vi "HandleObservationSync_002.vi"(8 "error in (no error)":errorcluster, 11 "S4GUI in":refnum<class "S4GUI.lvclass">) -> (0 "error out":errorcluster, 3 "S4GUI out":refnum<class "S4GUI.lvclass">)   [LabVIEW 2018, in "S4GUI.lvclass"] (continued)
              n1509 = Equal?(x=w4372, y=w4362) -> (x = y?=w4370:bool)
              n1510 = call-dynamic "Read stopping.vi"("error in (no error)"=w4365, "Channel in"=w4367) -> ("error out"=w4364:errorcluster, "stopping"=w4363:bool, "Channel out"=w4366:refnum<class "Channel.lvclass">)  [unwired: 7 in]
              n1511 = call-dynamic "Write Channel.vi"("error in (no error)"=w4364, "Channel.lvclass"=w4366, "Acquisition in"=w4375) -> ("error out"=w4377:errorcluster, "Acquisition out"=w4376:refnum<class "Acquisition.lvclass">)  [unwired: 7 in]
            }
          }
          n1512 = call-dynamic "Write AcquisitionC.vi"("error in (no error)"=w4240, "Acquisition.lvclass"=w4238, "S4ACS_GUI in"=w4239) -> ("error out"=w4234:errorcluster, "S4ACS_GUI out"=w4235:refnum<class "S4GUI.lvclass">)  [unwired: 7 in]
          n1513 = call-dynamic "Read AcquisitionD.vi"("error in (no error)"=w4234, "S4ACS_GUI in"=w4235) -> ("error out"=w4218:errorcluster, "Acquisition.lvclass"=w4220:refnum<class "Acquisition.lvclass">, "S4ACS_GUI out"=w4241:refnum<class "S4GUI.lvclass">)  [unwired: 7 in]
          n1514 = call-dynamic "Read enabled.vi"("error in (no error)"=w4218, "Server in"=w4220) -> ("error out"=w4217:errorcluster, "enabled"=w4208:bool, "Server out"=w4219:refnum<class "Acquisition.lvclass">)  [unwired: 7 in]
          n1515 = case shown="True" w4208 {
            tunnel: [w4340 w4356] -> w4243
            tunnel: [w4339 w4355] -> w4242
            tunnel: w4219 -> [w4340 w4354]
            tunnel: w4217 -> [w4339 w4353]
            tunnel: [0 ("State") w4351] -> w4199
            tunnel: w4211 -> [_ w4350]
            tunnel: [TRUE w4349] -> w4209
            tunnel: [FALSE ("stopping") w4342] -> w4195
            frame False {
            }
            frame True {
              n1516 = call-dynamic "Read Channel.vi"("error in (no error)"=w4353, "Acquisition in"=w4354) -> ("error out"=w4348:errorcluster, "Channel.lvclass"=w4347:refnum<class "Channel.lvclass">, "Acquisition out"=w4352:refnum<class "Acquisition.lvclass">)  [unwired: 7 in]
              n1517 = call-dynamic "Read CyclesDone.vi"("error in (no error)"=w4348, "Channel in"=w4347) -> ("error out"=w4344:errorcluster, "CyclesDone"=w4351:u32, "Channel out"=w4346:refnum<class "Channel.lvclass">)  [unwired: 7 in]
              n1518 = Increment(x=w4350) -> (x+1=w4341:u32)
              n1519 = Equal?(x=w4351, y=w4341) -> (x = y?=w4349:bool)
              n1520 = call-dynamic "Read stopping.vi"("error in (no error)"=w4344, "Channel in"=w4346) -> ("error out"=w4343:errorcluster, "stopping"=w4342:bool, "Channel out"=w4345:refnum<class "Channel.lvclass">)  [unwired: 7 in]
              n1521 = call-dynamic "Write Channel.vi"("error in (no error)"=w4343, "Channel.lvclass"=w4345, "Acquisition in"=w4352) -> ("error out"=w4355:errorcluster, "Acquisition out"=w4356:refnum<class "Acquisition.lvclass">)  [unwired: 7 in]
            }
          }
          n1522 = Build Array(w4207, w4206, w4205, w4208) -> (w4204:bool[])
          n1523 = Boolean Array To Number(Boolean array=w4204) -> (number=w4203:u32)
          n1524 = Max & Min(x=w4200, y=w4199) -> (max(x,y)=w4213:u32)  [unwired: 1 out]
          n1525 = Compound Arithmetic op=AND(w4215, w4212, w4210, w4209) -> (w4194:bool)
          n1526 = case shown="15" w4203 {
            tunnel: w4202 -> [w4292 _ w4304 _ w4313 _ w4319 w4325 _ w4331 w4334 _]
            tunnel: w4199 -> [w4291 w4295 w4300 w4307 w4308 w4316 w4318 _ _ _ _ _]
            tunnel: w4201 -> [w4290 w4293 _ _ w4312 w4314 _ w4324 w4328 _ w4333 _]
            tunnel: w4200 -> [w4289 w4294 w4299 w4305 _ _ _ w4323 w4327 w4330 _ _]
            tunnel: [w4285 w4296 w4301 w4306 w4309 w4315 w4317 w4320 w4326 w4329 w4332 TRUE] -> _
            frame 15 {
              # "A,B,C,D ativos"
              n1527 = Equal?(x=w4292, y=w4290) -> (x = y?=w4288:bool)
              n1528 = Equal?(x=w4289, y=w4291) -> (x = y?=w4286:bool)
              n1529 = Equal?(x=w4290, y=w4289) -> (x = y?=w4287:bool)
              n1530 = Compound Arithmetic op=AND(w4288, w4287, w4286) -> (w4285:bool)
            }
            frame 14 {
              # "B,C e,D ativos"
              n1531 = Equal?(x=w4293, y=w4294) -> (x = y?=w4298:bool)
              n1532 = Equal?(x=w4294, y=w4295) -> (x = y?=w4297:bool)
              n1533 = Compound Arithmetic op=AND(w4298, w4297) -> (w4296:bool)
            }
            frame 13 {
              # "A,C e,D ativos"
              n1534 = Equal?(x=w4304, y=w4299) -> (x = y?=w4303:bool)
              n1535 = Equal?(x=w4299, y=w4300) -> (x = y?=w4302:bool)
              n1536 = Compound Arithmetic op=AND(w4303, w4302) -> (w4301:bool)
            }
            frame 12 {
              # "Só C e D ativos"
              n1537 = Equal?(x=w4305, y=w4307) -> (x = y?=w4306:bool)
            }
            frame 11 {
              # "A,B e,D ativos"
              n1538 = Equal?(x=w4313, y=w4312) -> (x = y?=w4311:bool)
              n1539 = Equal?(x=w4312, y=w4308) -> (x = y?=w4310:bool)
              n1540 = Compound Arithmetic op=AND(w4311, w4310) -> (w4309:bool)
            }
            frame 10 {
              # "Só B e D ativos"
              n1541 = Equal?(x=w4314, y=w4316) -> (x = y?=w4315:bool)
            }
            frame 9 {
              # "Só A e D ativos"
              n1542 = Equal?(x=w4319, y=w4318) -> (x = y?=w4317:bool)
            }
            frame 7 {
              # "A,B,C ativos"
              n1543 = Equal?(x=w4325, y=w4324) -> (x = y?=w4322:bool)
              n1544 = Equal?(x=w4324, y=w4323) -> (x = y?=w4321:bool)
              n1545 = Compound Arithmetic op=AND(w4322, w4321) -> (w4320:bool)
            }
            frame 6 {
              # "Só B e C ativos"
              n1546 = Equal?(x=w4328, y=w4327) -> (x = y?=w4326:bool)
            }
            frame 5 {
              # "Só A e C ativos"
              n1547 = Equal?(x=w4331, y=w4330) -> (x = y?=w4329:bool)
            }
            frame 3 {
              # "só A e B ativos"
              n1548 = Equal?(x=w4334, y=w4333) -> (x = y?=w4332:bool)
            }
            frame 0..2, 4, 8, Default {
              # "nenhum ou só 1  \ncanal ativo."
            }
          }
          n1549 = Max & Min(x=w4214, y=w4213) -> (max(x,y)=w4192:u32)  [unwired: 1 out]
          n1550 = Compound Arithmetic op=OR(w4198, w4197, w4196, w4195) -> (w4193:bool)
          n1551 = call-dynamic "Write AcquisitionD.vi"("error in (no error)"=w4242, "Acquisition.lvclass"=w4243, "S4ACS_GUI in"=w4241) -> ("error out"=w4233:errorcluster, "S4ACS_GUI out"=w4190:refnum<class "S4GUI.lvclass">)  [unwired: 7 in]
          n1552 = case shown="True" w4194 {
            tunnel: w4190 -> [w4255 w4273]
            tunnel: [w4261 w4272] -> w4189
            tunnel: w4193 -> [_ w4274]
            tunnel: w4192 -> [_ w4271]
            tunnel: w4191 -> [w4253 w4270]
            frame False {
              # "Aguardando iniciar exposição por 5s"
              n1553 = local read "time1"() -> (w4254:u32)
              n1554 = Tick Count (ms)() -> (millisecond timer value=w4260:u32)
              n1555 = Subtract(x=w4260, y=w4254) -> (x-y=w4257:u32)
              n1556 = To Double Precision Float(number=w4257) -> (double precision float=w4259:dbl)
              n1557 = Less?(x=5000.0 ("y"), y=w4259) -> (x < y?=w4258:bool)
              n1558 = case shown="True" w4258 {
                tunnel: w4255 -> [w4265 w4269]
                tunnel: [w4264 w4268] -> w4261
                tunnel: w4253 -> [w4263 _]
                frame False {
                  # "Volta para esperar ACTIVE."
                  n1559 = Decrement(x=w4263) -> (x-1=w4262:u32)
                  n1560 = Bundle By Name(cluster=w4265, "Obs_state"=w4262) -> (w4264:refnum<class "S4GUI.lvclass">)
                }
                frame True {
                  n1561 = Bundle By Name(cluster=w4269, "Obs_state"=u32 1, "Error Msg"="ERROR: Init Acquisition Timeout. HandleObservationSync.vi - state 327.") -> (w4268:refnum<class "S4GUI.lvclass">)
                }
              }
            }
            frame True {
              # "STOP?"
              # "CIclo Avançou."
              n1562 = case shown="False" w4274 {
                tunnel: w4273 -> [w4278 w4284]
                tunnel: [w4277 w4283] -> w4272
                tunnel: w4271 -> [w4276 w4282]
                tunnel: w4270 -> [_ w4281]
                frame True {
                  # "STOP acionado."
                  n1563 = Bundle By Name(cluster=w4278, "Obs_state"=u32 0, "cyclesDone"=w4276) -> (w4277:refnum<class "S4GUI.lvclass">)
                }
                frame False {
                  # "Vai esperar fim da exposição..."
                  n1564 = Increment(x=w4281) -> (x+1=w4280:u32)
                  n1565 = Increment(x=w4280) -> (x+1=w4279:u32)
                  n1566 = Bundle By Name(cluster=w4284, "Obs_state"=w4279, "cyclesDone"=w4282) -> (w4283:refnum<class "S4GUI.lvclass">)
                }
              }
            }
          }
        }
        frame 328 {
          # "T= canais receberam STOP"
          n1567 = Unbundle By Name(w4444) -> ("cyclesDone"=w4438:u32)
          n1568 = call-dynamic "Read AcquisitionA.vi"("error in (no error)"=w4480, "S4ACS_GUI in"=w4444) -> ("error out"=w4459:errorcluster, "Acquisition.lvclass"=w4460:refnum<class "Acquisition.lvclass">, "S4ACS_GUI out"=w4482:refnum<class "S4GUI.lvclass">)  [unwired: 7 in]
          n1569 = call-dynamic "Read enabled.vi"("error in (no error)"=w4459, "Server in"=w4460) -> ("error out"=w4458:errorcluster, "enabled"=w4434:bool, "Server out"=w4457:refnum<class "Acquisition.lvclass">)  [unwired: 7 in]
          n1570 = case shown="True" w4434 {
            tunnel: w4458 -> [w4631 w4648]
            tunnel: [w4632 w4646] -> w4483
            tunnel: [w4631 w4645] -> w4481
            tunnel: [0 ("State") w4641] -> w4429
            tunnel: w4457 -> [w4632 w4640]
            tunnel: w4438 -> [_ w4639]
            tunnel: [TRUE w4638] -> w4443
            tunnel: [FALSE ("stopping") w4634] -> w4425
            frame False {
            }
            frame True {
              n1571 = call-dynamic "Read Channel.vi"("error in (no error)"=w4648, "Acquisition in"=w4640) -> ("error out"=w4644:errorcluster, "Channel.lvclass"=w4643:refnum<class "Channel.lvclass">, "Acquisition out"=w4647:refnum<class "Acquisition.lvclass">)  [unwired: 7 in]
              n1572 = call-dynamic "Read CyclesDone.vi"("error in (no error)"=w4644, "Channel in"=w4643) -> ("error out"=w4636:errorcluster, "CyclesDone"=w4641:u32, "Channel out"=w4642:refnum<class "Channel.lvclass">)  [unwired: 7 in]
              n1573 = Increment(x=w4639) -> (x+1=w4633:u32)
              n1574 = Equal?(x=w4641, y=w4633) -> (x = y?=w4638:bool)
              n1575 = call-dynamic "Read stopping.vi"("error in (no error)"=w4636, "Channel in"=w4642) -> ("error out"=w4635:errorcluster, "stopping"=w4634:bool, "Channel out"=w4637:refnum<class "Channel.lvclass">)  [unwired: 7 in]
              n1576 = call-dynamic "Write Channel.vi"("error in (no error)"=w4635, "Channel.lvclass"=w4637, "Acquisition in"=w4647) -> ("error out"=w4645:errorcluster, "Acquisition out"=w4646:refnum<class "Acquisition.lvclass">)  [unwired: 7 in]
            }
          }
          n1577 = call-dynamic "Write AcquisitionA.vi"("error in (no error)"=w4481, "Acquisition.lvclass"=w4483, "S4ACS_GUI in"=w4482) -> ("error out"=w4476:errorcluster, "S4ACS_GUI out"=w4475:refnum<class "S4GUI.lvclass">)  [unwired: 7 in]
          n1578 = call "Read AcquisitionB.vi"("error in (no error)"=w4476, "S4ACS_GUI in"=w4475) -> ("error out"=w4453:errorcluster, "Acquisition.lvclass"=w4456:refnum<class "Acquisition.lvclass">, "S4ACS_GUI out"=w4477:refnum<class "S4GUI.lvclass">)  [unwired: 7 in]
          n1579 = call-dynamic "Read enabled.vi"("error in (no error)"=w4453, "Server in"=w4456) -> ("error out"=w4454:errorcluster, "enabled"=w4433:bool, "Server out"=w4455:refnum<class "Acquisition.lvclass">)  [unwired: 7 in]
          n1580 = case shown="True" w4433 {
            tunnel: w4454 -> [w4610 w4627]
            tunnel: w4455 -> [w4611 w4626]
            tunnel: [0 ("State") w4619] -> w4428
            tunnel: [w4610 w4625] -> w4474
            tunnel: [w4611 w4624] -> w4473
            tunnel: w4438 -> [_ w4618]
            tunnel: [TRUE w4617] -> w4439
            tunnel: [FALSE ("stopping") w4613] -> w4424
            frame False {
            }
            frame True {
              n1581 = call-dynamic "Read Channel.vi"("error in (no error)"=w4627, "Acquisition in"=w4626) -> ("error out"=w4622:errorcluster, "Channel.lvclass"=w4623:refnum<class "Channel.lvclass">, "Acquisition out"=w4620:refnum<class "Acquisition.lvclass">)  [unwired: 7 in]
              n1582 = call-dynamic "Read CyclesDone.vi"("error in (no error)"=w4622, "Channel in"=w4623) -> ("error out"=w4615:errorcluster, "CyclesDone"=w4619:u32, "Channel out"=w4621:refnum<class "Channel.lvclass">)  [unwired: 7 in]
              n1583 = Increment(x=w4618) -> (x+1=w4612:u32)
              n1584 = Equal?(x=w4619, y=w4612) -> (x = y?=w4617:bool)
              n1585 = call-dynamic "Read stopping.vi"("error in (no error)"=w4615, "Channel in"=w4621) -> ("error out"=w4614:errorcluster, "stopping"=w4613:bool, "Channel out"=w4616:refnum<class "Channel.lvclass">)  [unwired: 7 in]
              n1586 = call-dynamic "Write Channel.vi"("error in (no error)"=w4614, "Channel.lvclass"=w4616, "Acquisition in"=w4620) -> ("error out"=w4625:errorcluster, "Acquisition out"=w4624:refnum<class "Acquisition.lvclass">)  [unwired: 7 in]
            }
          }
          n1587 = Max & Min(x=w4429, y=w4428) -> (max(x,y)=w4442:u32)  [unwired: 1 out]
          n1588 = call "Write AcquisitionB.vi"("error in (no error)"=w4474, "Acquisition.lvclass"=w4473, "S4ACS_GUI in"=w4477) -> ("error out"=w4466:errorcluster, "S4ACS_GUI out"=w4465:refnum<class "S4GUI.lvclass">)  [unwired: 7 in]
          n1589 = call-dynamic "Read AcquisitionC.vi"("error in (no error)"=w4466, "S4ACS_GUI in"=w4465) -> ("error out"=w4450:errorcluster, "Acquisition.lvclass"=w4452:refnum<class "Acquisition.lvclass">, "S4ACS_GUI out"=w4468:refnum<class "S4GUI.lvclass">)  [unwired: 7 in]
          n1590 = call-dynamic "Read enabled.vi"("error in (no error)"=w4450, "Server in"=w4452) -> ("error out"=w4449:errorcluster, "enabled"=w4432:bool, "Server out"=w4451:refnum<class "Acquisition.lvclass">)  [unwired: 7 in]
          n1591 = case shown="True" w4432 {
            tunnel: [w4589 w4606] -> w4469
            tunnel: [w4590 w4605] -> w4467
            tunnel: w4449 -> [w4589 w4602]
            tunnel: w4451 -> [w4590 w4603]
            tunnel: [0 ("State") w4601] -> w4427
            tunnel: w4438 -> [_ w4600]
            tunnel: [TRUE w4599] -> w4437
            tunnel: [FALSE ("stopping") w4592] -> w4423
            frame False {
            }
            frame True {
              n1592 = call-dynamic "Read Channel.vi"("error in (no error)"=w4602, "Acquisition in"=w4603) -> ("error out"=w4598:errorcluster, "Channel.lvclass"=w4597:refnum<class "Channel.lvclass">, "Acquisition out"=w4604:refnum<class "Acquisition.lvclass">)  [unwired: 7 in]
              n1593 = call-dynamic "Read CyclesDone.vi"("error in (no error)"=w4598, "Channel in"=w4597) -> ("error out"=w4594:errorcluster, "CyclesDone"=w4601:u32, "Channel out"=w4596:refnum<class "Channel.lvclass">)  [unwired: 7 in]
              n1594 = Increment(x=w4600) -> (x+1=w4591:u32)
              n1595 = Equal?(x=w4601, y=w4591) -> (x = y?=w4599:bool)
              n1596 = call-dynamic "Read stopping.vi"("error in (no error)"=w4594, "Channel in"=w4596) -> ("error out"=w4593:errorcluster, "stopping"=w4592:bool, "Channel out"=w4595:refnum<class "Channel.lvclass">)  [unwired: 7 in]
              n1597 = call-dynamic "Write Channel.vi"("error in (no error)"=w4593, "Channel.lvclass"=w4595, "Acquisition in"=w4604) -> ("error out"=w4606:errorcluster, "Acquisition out"=w4605:refnum<class "Acquisition.lvclass">)  [unwired: 7 in]
            }
          }
          n1598 = call-dynamic "Write AcquisitionC.vi"("error in (no error)"=w4469, "Acquisition.lvclass"=w4467, "S4ACS_GUI in"=w4468) -> ("error out"=w4463:errorcluster, "S4ACS_GUI out"=w4464:refnum<class "S4GUI.lvclass">)  [unwired: 7 in]
          n1599 = call-dynamic "Read AcquisitionD.vi"("error in (no error)"=w4463, "S4ACS_GUI in"=w4464) -> ("error out"=w4446:errorcluster, "Acquisition.lvclass"=w4448:refnum<class "Acquisition.lvclass">, "S4ACS_GUI out"=w4470:refnum<class "S4GUI.lvclass">)  [unwired: 7 in]
          n1600 = call-dynamic "Read enabled.vi"("error in (no error)"=w4446, "Server in"=w4448) -> ("error out"=w4445:errorcluster, "enabled"=w4435:bool, "Server out"=w4447:refnum<class "Acquisition.lvclass">)  [unwired: 7 in]
          n1601 = case shown="True" w4435 {
            tunnel: [w4569 w4585] -> w4472
            tunnel: [w4568 w4584] -> w4471
            tunnel: w4447 -> [w4569 w4583]
            tunnel: w4445 -> [w4568 w4582]
            tunnel: [0 ("State") w4580] -> w4426
            tunnel: w4438 -> [_ w4579]
            tunnel: [TRUE w4578] -> w4436
            tunnel: [FALSE ("stopping") w4571] -> w4422
            frame False {
            }
            frame True {
              n1602 = call-dynamic "Read Channel.vi"("error in (no error)"=w4582, "Acquisition in"=w4583) -> ("error out"=w4577:errorcluster, "Channel.lvclass"=w4576:refnum<class "Channel.lvclass">, "Acquisition out"=w4581:refnum<class "Acquisition.lvclass">)  [unwired: 7 in]
              n1603 = call-dynamic "Read CyclesDone.vi"("error in (no error)"=w4577, "Channel in"=w4576) -> ("error out"=w4573:errorcluster, "CyclesDone"=w4580:u32, "Channel out"=w4575:refnum<class "Channel.lvclass">)  [unwired: 7 in]
              n1604 = Increment(x=w4579) -> (x+1=w4570:u32)
              n1605 = Equal?(x=w4580, y=w4570) -> (x = y?=w4578:bool)
              n1606 = call-dynamic "Read stopping.vi"("error in (no error)"=w4573, "Channel in"=w4575) -> ("error out"=w4572:errorcluster, "stopping"=w4571:bool, "Channel out"=w4574:refnum<class "Channel.lvclass">)  [unwired: 7 in]
              n1607 = call-dynamic "Write Channel.vi"("error in (no error)"=w4572, "Channel.lvclass"=w4574, "Acquisition in"=w4581) -> ("error out"=w4584:errorcluster, "Acquisition out"=w4585:refnum<class "Acquisition.lvclass">)  [unwired: 7 in]
            }
          }
          n1608 = Build Array(w4434, w4433, w4432, w4435) -> (w4431:bool[])
          n1609 = Boolean Array To Number(Boolean array=w4431) -> (number=w4430:u32)
          n1610 = Max & Min(x=w4427, y=w4426) -> (max(x,y)=w4441:u32)  [unwired: 1 out]
          n1611 = Compound Arithmetic op=AND(w4443, w4439, w4437, w4436) -> (w4420:bool)
          n1612 = case shown="15" w4430 {
            tunnel: w4429 -> [w4491 _ w4503 _ w4512 _ w4518 w4524 _ w4530 w4533 _]
            tunnel: w4426 -> [w4490 w4494 w4499 w4506 w4507 w4515 w4517 _ _ _ _ _]
            tunnel: w4428 -> [w4489 w4492 _ _ w4511 w4513 _ w4523 w4527 _ w4532 _]
            tunnel: w4427 -> [w4488 w4493 w4498 w4504 _ _ _ w4522 w4526 w4529 _ _]
            tunnel: [w4484 w4495 w4500 w4505 w4508 w4514 w4516 w4519 w4525 w4528 w4531 TRUE] -> _
            frame 15 {
              # "A,B,C,D ativos"
              n1613 = Equal?(x=w4491, y=w4489) -> (x = y?=w4487:bool)
              n1614 = Equal?(x=w4488, y=w4490) -> (x = y?=w4485:bool)
              n1615 = Equal?(x=w4489, y=w4488) -> (x = y?=w4486:bool)
              n1616 = Compound Arithmetic op=AND(w4487, w4486, w4485) -> (w4484:bool)
            }
            frame 14 {
              # "B,C e,D ativos"
              n1617 = Equal?(x=w4492, y=w4493) -> (x = y?=w4497:bool)
              n1618 = Equal?(x=w4493, y=w4494) -> (x = y?=w4496:bool)
              n1619 = Compound Arithmetic op=AND(w4497, w4496) -> (w4495:bool)
            }
            frame 13 {
              # "A,C e,D ativos"
              n1620 = Equal?(x=w4503, y=w4498) -> (x = y?=w4502:bool)
              n1621 = Equal?(x=w4498, y=w4499) -> (x = y?=w4501:bool)
              n1622 = Compound Arithmetic op=AND(w4502, w4501) -> (w4500:bool)
            }
            frame 12 {
              # "Só C e D ativos"
              n1623 = Equal?(x=w4504, y=w4506) -> (x = y?=w4505:bool)
            }
            frame 11 {
              # "A,B e,D ativos"
              n1624 = Equal?(x=w4512, y=w4511) -> (x = y?=w4510:bool)
              n1625 = Equal?(x=w4511, y=w4507) -> (x = y?=w4509:bool)
              n1626 = Compound Arithmetic op=AND(w4510, w4509) -> (w4508:bool)
            }
            frame 10 {
              # "Só B e D ativos"
              n1627 = Equal?(x=w4513, y=w4515) -> (x = y?=w4514:bool)
            }
            frame 9 {
              # "Só A e D ativos"
              n1628 = Equal?(x=w4518, y=w4517) -> (x = y?=w4516:bool)
            }
            frame 7 {
              # "A,B,C ativos"
              n1629 = Equal?(x=w4524, y=w4523) -> (x = y?=w4521:bool)
              n1630 = Equal?(x=w4523, y=w4522) -> (x = y?=w4520:bool)
              n1631 = Compound Arithmetic op=AND(w4521, w4520) -> (w4519:bool)
            }
            frame 6 {
              # "Só B e C ativos"
              n1632 = Equal?(x=w4527, y=w4526) -> (x = y?=w4525:bool)
            }
            frame 5 {
              # "Só A e C ativos"
              n1633 = Equal?(x=w4530, y=w4529) -> (x = y?=w4528:bool)
            }
            frame 3 {
              # "só A e B ativos"
              n1634 = Equal?(x=w4533, y=w4532) -> (x = y?=w4531:bool)
            }
            frame 0..2, 4, 8, Default {
              # "nenhum ou só 1  \ncanal ativo."
            }
          }
          n1635 = Max & Min(x=w4442, y=w4441) -> (max(x,y)=w4440:u32)  [unwired: 1 out]
          n1636 = Compound Arithmetic op=OR(w4425, w4424, w4423, w4422) -> (w4421:bool)
          n1637 = call-dynamic "Write AcquisitionD.vi"("error in (no error)"=w4471, "Acquisition.lvclass"=w4472, "S4ACS_GUI in"=w4470) -> ("error out"=w4461:errorcluster, "S4ACS_GUI out"=w4462:refnum<class "S4GUI.lvclass">)  [unwired: 7 in]
          n1638 = case shown="True" w4420 {
            tunnel: w4462 -> [w4545 w4555]
            tunnel: [w4544 w4554] -> w4479
            tunnel: w4478 -> [_ w4553]
            tunnel: w4440 -> [_ w4552]
            tunnel: w4421 -> [_ w4551]
            frame False {
              # "Aguardando avanço do ciclo."
              n1639 = local read "time307"() -> (w4535:u32)
              n1640 = Tick Count (ms)() -> (millisecond timer value=w4543:u32)
              n1641 = Subtract(x=w4543, y=w4535) -> (x-y=w4540:u32)
              n1642 = call-dynamic "GetGreatestCube.vi"("S4GUI in"=w4545) -> ("S4GUI out"=w4536:refnum<class "S4GUI.lvclass">, "greatest (ms)"=w4538:dbl)  [unwired: 8 in, 1 out]
              n1643 = To Double Precision Float(number=w4540) -> (double precision float=w4542:dbl)
              n1644 = Add(x=5000.0 ("y"), y=w4538) -> (x+y=w4537:dbl)
              n1645 = Less?(x=w4537, y=w4542) -> (x < y?=w4541:bool)
              n1646 = case shown="True" w4541 {
                tunnel: w4536 -> [w4546 w4550]
                tunnel: [w4546 w4549] -> w4544
                frame False {
                }
                frame True {
                  n1647 = Bundle By Name(cluster=w4550, "Obs_state"=u32 1, "Error Msg"="ERROR: Acquisition Timeout. HandleObservationSync.vi - state 328.") -> (w4549:refnum<class "S4GUI.lvclass">)
                }
              }
            }
            frame True {
              # "Ciclo avançou."
              # "STOP?"
              n1648 = case shown="False" w4551 {
                tunnel: w4555 -> [w4559 w4564]
                tunnel: [w4558 w4563] -> w4554
                tunnel: w4553 -> [_ w4561]
                tunnel: w4552 -> [w4557 w4560]
                frame True {
                  n1649 = Bundle By Name(cluster=w4559, "Obs_state"=u32 0, "cyclesDone"=w4557) -> (w4558:refnum<class "S4GUI.lvclass">)
                }
                frame False {
                  n1650 = Increment(x=w4561) -> (x+1=w4562:u32)
                  n1651 = Bundle By Name(cluster=w4564, "Obs_state"=w4562, "cyclesDone"=w4560) -> (w4563:refnum<class "S4GUI.lvclass">)
                }
              }
            }
          }
        }
        frame 329 {
          n1652 = disable-structure shown="Enabled" {
            disable-tunnel: w4653 -> [w4667 w4673]
            disable-tunnel: w4652 -> [w4666 w4680]
            disable-tunnel: [w4665 w4680] -> w4651
            disable-tunnel: [w4663 w4681] -> w4650
            disable-tunnel: w4649 -> [_ w4674]
            frame Disabled {
              n1653 = call-dynamic "Read ciclos.vi"("error in (no error)"=w4666, "S4ACS_GUI in"=w4667) -> ("error out"=w4655:errorcluster, "ciclos"=w4660:u32, "S4ACS_GUI out"=w4668:refnum<class "S4GUI.lvclass">)  [unwired: 7 in]
              n1654 = Decrement(x=w4660) -> (x-1=w4654:u32)
              n1655 = Greater Than 0?(x=w4654) -> (x > 0?=w4661:bool)
              n1656 = case shown="False" w4661 {
                selector: w4661 -> [w4670 w4672]
                tunnel: w4654 -> [_ w4671]
                tunnel: [w4670 w4672] -> w4659
                tunnel: [u32 0 w4671] -> w4656
                frame False {
                }
                frame True {
                }
              }
              n1657 = Select(t=u32 323, s=w4659, f=u32 0) -> (s? t:f=w4662:u32)
              n1658 = call-dynamic "Write ciclos.vi"("error in (no error)"=w4655, "ciclos"=w4656, "S4ACS_GUI in"=w4668) -> ("error out"=w4665:errorcluster, "S4ACS_GUI out"=w4664:refnum<class "S4GUI.lvclass">)  [unwired: 7 in]
              n1659 = Bundle By Name(cluster=w4664, "Obs_state"=w4662) -> (w4663:refnum<class "S4GUI.lvclass">)
            }
            frame Enabled {
              n1660 = Unbundle By Name(w4673) -> ("TotalCiclos"=w4683:u32, "cyclesDone"=w4682:u32)
              n1661 = Subtract(x=w4683, y=w4682) -> (x-y=w4676:u32)
              n1662 = Greater Than 0?(x=w4676) -> (x > 0?=w4679:bool)
              n1663 = disable-structure shown="Enabled" {
                disable-tunnel: [w4685 u32 325 ("t")] -> w4675
                disable-tunnel: w4674 -> [w4684 _]
                frame Disabled {
                  n1664 = Increment(x=w4684) -> (x+1=w4685:u32)
                }
                frame Enabled {
                }
              }
              n1665 = Select(t=w4675, s=w4679, f=u32 0) -> (s? t:f=w4678:u32)
              n1666 = Bundle By Name(cluster=w4673, "ciclos"=w4676, "Obs_state"=w4678) -> (w4681:refnum<class "S4GUI.lvclass">)
            }
          }
        }
        frame 350 {
          n1667 = flat-sequence {
            tunnel: w4688 -> [w4728]
            tunnel: [w4728] -> w4687
            frame #0 {
              n1668 = Tick Count (ms)() -> (millisecond timer value=→"timer350":u32)
            }
          }
          n1669 = call "Read Instrument.lvclass.vi"("error in (no error)"=w4687, "S4ACS_GUI in"=w4723) -> ("error out"=w4726:errorcluster, "Instrument.lvclass"=w4727:refnum<class "Instrument.lvclass">, "S4ACS_GUI out"=w4724:refnum<class "S4GUI.lvclass">)  [unwired: 7 in]
          n1670 = call "Read WPROT.vi"("error in (no error)"=w4726, "Instrument in"=w4727) -> ("error out"=w4716:errorcluster, "Opt_Selector.lvclass"=w4717:refnum<class "Opt_Selector.lvclass">, "Instrument out"=w4725:refnum<class "Instrument.lvclass">)  [unwired: 7 in]
          n1671 = call-dynamic "getTargetPos.vi"("error in (no error)"=w4716, "Opt_Selector in"=w4717) -> ("error out"=w4715:errorcluster, "Target Pos"=w4695:u16, "Opt_Selector out"=w4714:refnum<class "Opt_Selector.lvclass">)  [unwired: 7 in]
          n1672 = Build Array(-1.0 ("element"), 0.0 ("element"), 22.5 ("element"), 45.0 ("element"), 67.5 ("element"), 90.0 ("element"), 112.5 ("element"), 135.0 ("element"), 157.5 ("element"), 180.0 ("element"), 202.5 ("element"), 225.0 ("element"), 247.5 ("element"), 270.0 ("element"), 292.5 ("element"), 315.0 ("element"), 337.5 ("element")) -> (w4707:dbl[])
          n1673 = Index Array(array=w4707, index=w4695) -> (element=w4694:dbl)
          n1674 = case shown="0, Default" w4695 {
            selector: w4695 -> [_ w4757]
            tunnel: w4725 -> [w4737 w4745]
            tunnel: [w4737 w4745] -> w4690
            tunnel: [w4734 w4744] -> w4689
            tunnel: w4720 -> [_ w4759]
            tunnel: [u32 352 w4758] -> w4719
            tunnel: w4715 -> [w4735 w4753]
            tunnel: w4714 -> [w4736 w4752]
            tunnel: w4694 -> [_ w4747]
            tunnel: [w4732 w4746] -> w4691
            frame 0, Default {
              # "Terminou uma sequência.\nRecupera as posições em SEQ e desvia para 311 para verificar se há mais ciclos."
              # "Recupera a sequencia anterior para o caso \nde repetição da sequencia (sem precisar clicar \nnas posicoes desejadas novamente)."
              n1675 = call-dynamic "Read sequencia_ant.vi"("error in (no error)"=w4735, "Opt_Selector in"=w4736) -> ("error out"=w4731:errorcluster, "sequencia_ant"=w4730:u16, "Opt_Selector out"=w4733:refnum<class "Opt_Selector.lvclass">)  [unwired: 7 in]
              n1676 = call-dynamic "Write sequencia.vi"("error in (no error)"=w4731, "sequencia"=w4730, "Opt_Selector in"=w4733) -> ("error out"=w4734:errorcluster, "Opt_Selector out"=w4732:refnum<class "Opt_Selector.lvclass">)  [unwired: 7 in]
            }
            frame 1..16 {
              # "Espera até 40 x 0.25s (= 10s) para\nmecanismo entrar em READY"
              n1677 = Number To Decimal String(number=w4757) -> (decimal integer string=w4756:string)  [unwired: 1 in]
              n1678 = Concatenate Strings("WP" ("string"), w4756) -> (w4754:string)
              n1679 = call "Write target name.vi"("error in (no error)"=w4753, "target name"=w4754, "Optics in"=w4752) -> ("error out"=w4750:errorcluster, "Optics out"=w4751:refnum<class "Opt_Selector.lvclass">)  [unwired: 7 in]
              n1680 = call "Write target.vi"("error in (no error)"=w4750, "target"=w4747, "Optics in"=w4751) -> ("error out"=w4749:errorcluster, "Optics out"=w4748:refnum<class "Opt_Selector.lvclass">)  [unwired: 7 in]
              n1681 = call-dynamic "Read State Machine.vi"("error in (no error)"=w4749, "Device in"=w4748) -> ("error out"=w4761:errorcluster, "State Machine.lvclass"=w4763:refnum<class "State Machine.lvclass">, "Device out"=w4760:refnum<class "Opt_Selector.lvclass">)  [unwired: 7 in]
              n1682 = Increment(x=w4759) -> (x+1=w4758:u32)
              n1683 = call "Next State.vi"("error in (no error)"=w4761, "New_State"=1, "State Machine in"=w4763) -> ("error out"=w4741:errorcluster, "State Machine out"=w4743:refnum<class "State Machine.lvclass">)  [unwired: 7 in]
              n1684 = call-dynamic "Write Timer.vi"("error in (no error)"=w4741, "Timer"=u32 40, "State Machine in"=w4743) -> ("error out"=w4740:errorcluster, "State Machine out"=w4742:refnum<class "State Machine.lvclass">)  [unwired: 7 in]
              n1685 = call-dynamic "Write State Machine.vi"("error in (no error)"=w4740, "State Machine.lvclass"=w4742, "Device in"=w4760) -> ("error out"=w4744:errorcluster, "Device out"=w4746:refnum<class "Opt_Selector.lvclass">)  [unwired: 7 in]
            }
          }
          n1686 = call "Write WPROT.vi"("error in (no error)"=w4689, "Opt_Selector.lvclass"=w4691, "Instrument in"=w4690) -> ("error out"=w4693:errorcluster, "Instrument out"=w4692:refnum<class "Instrument.lvclass">)  [unwired: 7 in]
          n1687 = call "Write Instrument.lvclass.vi"("error in (no error)"=w4693, "Instrument.lvclass"=w4692, "S4ACS_GUI in"=w4724) -> ("error out"=w4722:errorcluster, "S4ACS_GUI out"=w4721:refnum<class "S4GUI.lvclass">)  [unwired: 7 in]
          n1688 = Bundle By Name(cluster=w4721, "Obs_state"=w4719) -> (w4718:refnum<class "S4GUI.lvclass">)
        }
        frame 351 {
          # "Espera terminar o movimento da lamina para disparar a aquisição\ndos canais ativos.\n\nOV 20230424: Não precisa mais atualizar o valor de WPPOS com o\ncomando WRITE_HEADER porque o ACS já recebeu a sequência de\nposições da lâmina."
          n1689 = flat-sequence {
            tunnel: w4774 -> [w4793]
            tunnel: [w4793] -> w4773
            frame #0 {
              n1690 = Tick Count (ms)() -> (millisecond timer value=w4792:u32)
              "timer351" <- w4792
              n1691 = local read "time1"() -> (w4791:u32)
              n1692 = Subtract(x=w4792, y=w4791) -> (x-y=→"delay wp 2":u32)
            }
          }
          n1693 = call "Read Instrument.lvclass.vi"("error in (no error)"=w4773, "S4ACS_GUI in"=w4783) -> ("error out"=w4788:errorcluster, "Instrument.lvclass"=w4789:refnum<class "Instrument.lvclass">, "S4ACS_GUI out"=w4785:refnum<class "S4GUI.lvclass">)  [unwired: 7 in]
          n1694 = call "Read WPROT.vi"("error in (no error)"=w4788, "Instrument in"=w4789) -> ("error out"=w4780:errorcluster, "Opt_Selector.lvclass"=w4779:refnum<class "Opt_Selector.lvclass">, "Instrument out"=w4787:refnum<class "Instrument.lvclass">)  [unwired: 7 in]
          n1695 = call-dynamic "Read State Machine.vi"("error in (no error)"=w4780, "Device in"=w4779) -> ("error out"=w4781:errorcluster, "State Machine.lvclass"=w4782:refnum<class "State Machine.lvclass">, "Device out"=w4777:refnum<class "Opt_Selector.lvclass">)  [unwired: 7 in]
          n1696 = call-dynamic "Read State.vi"("error in (no error)"=w4781, "State Machine in"=w4782) -> ("error out"=w4771:errorcluster, "State"=w4775:i32, "State Machine out"=w4772:refnum<class "State Machine.lvclass">)  [unwired: 7 in]
          n1697 = Equal To 0?(x=w4775) -> (x = 0?=w4766:bool)
          n1698 = call-dynamic "Write State Machine.vi"("error in (no error)"=w4771, "State Machine.lvclass"=w4772, "Device in"=w4777) -> ("error out"=w4776:errorcluster, "Device out"=w4778:refnum<class "Opt_Selector.lvclass">)  [unwired: 7 in]
          n1699 = call "Write WPROT.vi"("error in (no error)"=w4776, "Opt_Selector.lvclass"=w4778, "Instrument in"=w4787) -> ("error out"=w4784:errorcluster, "Instrument out"=w4786:refnum<class "Instrument.lvclass">)  [unwired: 7 in]
          n1700 = call "Write Instrument.lvclass.vi"("error in (no error)"=w4784, "Instrument.lvclass"=w4786, "S4ACS_GUI in"=w4785) -> ("error out"=w4764:errorcluster, "S4ACS_GUI out"=w4767:refnum<class "S4GUI.lvclass">)  [unwired: 7 in]
          n1701 = Select(t=u32 350, s=w4766, f=w4765) -> (s? t:f=w4770:u32)
          n1702 = Bundle By Name(cluster=w4767, "Obs_state"=w4770) -> (w4768:refnum<class "S4GUI.lvclass">)
        }
        frame 352 {
          n1703 = disable-structure shown="Enabled" {
            disable-tunnel: w4797 -> [w4811 w4824]
            disable-tunnel: w4796 -> [w4810 w4822]
            disable-tunnel: [w4809 w4822] -> w4795
            disable-tunnel: [w4807 w4823] -> w4794
            frame Disabled {
              n1704 = call-dynamic "Read ciclos.vi"("error in (no error)"=w4810, "S4ACS_GUI in"=w4811) -> ("error out"=w4799:errorcluster, "ciclos"=w4804:u32, "S4ACS_GUI out"=w4812:refnum<class "S4GUI.lvclass">)  [unwired: 7 in]
              n1705 = Decrement(x=w4804) -> (x-1=w4798:u32)
              n1706 = Greater Than 0?(x=w4798) -> (x > 0?=w4805:bool)
              n1707 = case shown="False" w4805 {
                selector: w4805 -> [w4814 w4816]
                tunnel: w4798 -> [_ w4815]
                tunnel: [w4814 w4816] -> w4803
                tunnel: [u32 0 w4815] -> w4800
                frame False {
                }
                frame True {
                }
              }
              n1708 = Select(t=u32 323, s=w4803, f=u32 0) -> (s? t:f=w4806:u32)
              n1709 = call-dynamic "Write ciclos.vi"("error in (no error)"=w4799, "ciclos"=w4800, "S4ACS_GUI in"=w4812) -> ("error out"=w4809:errorcluster, "S4ACS_GUI out"=w4808:refnum<class "S4GUI.lvclass">)  [unwired: 7 in]
              n1710 = Bundle By Name(cluster=w4808, "Obs_state"=w4806) -> (w4807:refnum<class "S4GUI.lvclass">)
            }
            frame Enabled {
              n1711 = Unbundle By Name(w4824) -> ("cycles wprot"=w4825:u32)
              n1712 = Decrement(x=w4825) -> (x-1=w4817:u32)
              n1713 = Greater Than 0?(x=w4817) -> (x > 0?=w4821:bool)
              n1714 = Select(t=u32 350, s=w4821, f=u32 0) -> (s? t:f=w4820:u32)
              n1715 = Bundle By Name(cluster=w4824, "Obs_state"=w4820, "cycles wprot"=w4817) -> (w4823:refnum<class "S4GUI.lvclass">)
            }
          }
        }
        frame 360 {
          w4826 = u32 0 ("cyclesDone")
          # "Inicia o Ticks com\nvalor do relogio atual"
          # "Espera até 40 x 0.25s (= 10s) para\nmecanismo entrar em READY"
          # "Busca próximo valor de foco..."
          n1716 = flat-sequence {
            tunnel: w4843 -> [w4858]
            tunnel: [w4858] -> w4842
            frame #0 {
              n1717 = Tick Count (ms)() -> (millisecond timer value=→"time7":u32)
            }
          }
          n1718 = call-dynamic "Read TelFocus.lvclass.vi"("error in (no error)"=w4842, "S4GUI in"=w4854) -> ("error out"=w4856:errorcluster, "TelFocus.lvclass"=w4857:refnum<class "TelFocus.lvclass">, "S4GUI out"=w4855:refnum<class "S4GUI.lvclass">)  [unwired: 7 in]
          n1719 = call-dynamic "GetNextFocus.vi"("error in (no error)"=w4856, "TelFocus in"=w4857) -> ("error out"=w4840:errorcluster, "TelFocus out"=w4841:refnum<class "TelFocus.lvclass">)  [unwired: 8 in]
          n1720 = call-dynamic "Read SecMirror.lvclass.vi"("error in (no error)"=w4840, "TelFocus in"=w4841) -> ("error out"=w4827:errorcluster, "SecMirror.lvclass"=w4828:refnum<class "SecMirror.lvclass">, "TelFocus out"=w4845:refnum<class "TelFocus.lvclass">)  [unwired: 7 in]
          n1721 = call-dynamic "Read State Machine.vi"("error in (no error)"=w4827, "Device in"=w4828) -> ("error out"=w4837:errorcluster, "State Machine.lvclass"=w4839:refnum<class "State Machine.lvclass">, "Device out"=w4836:refnum<class "SecMirror.lvclass">)  [unwired: 7 in]
          n1722 = call "Next State.vi"("error in (no error)"=w4837, "New_State"=1, "State Machine in"=w4839) -> ("error out"=w4834:errorcluster, "State Machine out"=w4835:refnum<class "State Machine.lvclass">)  [unwired: 7 in]
          n1723 = call-dynamic "Write Timer.vi"("error in (no error)"=w4834, "Timer"=u32 40, "State Machine in"=w4835) -> ("error out"=w4831:errorcluster, "State Machine out"=w4832:refnum<class "State Machine.lvclass">)  [unwired: 7 in]
          n1724 = call-dynamic "Init Ticks2.vi"("error in (no error)"=w4831, "State Machine in"=w4832) -> ("error out"=w4830:errorcluster, "State Machine out"=w4829:refnum<class "State Machine.lvclass">)  [unwired: 8 in]
          n1725 = call-dynamic "Write State Machine.vi"("error in (no error)"=w4830, "State Machine.lvclass"=w4829, "Device in"=w4836) -> ("error out"=w4844:errorcluster, "Device out"=w4846:refnum<class "SecMirror.lvclass">)  [unwired: 7 in]
          n1726 = call-dynamic "Write SecMirror.lvclass.vi"("error in (no error)"=w4844, "SecMirror.lvclass"=w4846, "TelFocus in"=w4845) -> ("error out"=w4848:errorcluster, "TelFocus out"=w4847:refnum<class "TelFocus.lvclass">)  [unwired: 7 in]
          n1727 = call-dynamic "Write TelFocus.lvclass.vi"("error in (no error)"=w4848, "TelFocus.lvclass"=w4847, "S4GUI in"=w4855) -> ("error out"=w4853:errorcluster, "S4GUI out"=w4852:refnum<class "S4GUI.lvclass">)  [unwired: 7 in]
          n1728 = Increment(x=w4851) -> (x+1=w4850:u32)
          n1729 = Bundle By Name(cluster=w4852, "Obs_state"=w4850, "cyclesDone"=w4826, "sequesDone"=w4826) -> (w4849:refnum<class "S4GUI.lvclass">)
        }
        frame 361 {
          # "90: estado de erro."
          # "Timeout= 25s + distancia do target (cada 1000um=1s)"
          # "Espera terminar o movimento do foco do 2ndario para \ndisparar a aquisição do canal."
          n1730 = flat-sequence {
            tunnel: w4898 -> [w4920]
            tunnel: [w4920] -> w4897
            frame #0 {
              n1731 = Tick Count (ms)() -> (millisecond timer value=w4919:u32)
              "time 8" <- w4919
              n1732 = local read "time1"() -> (w4918:u32)
              n1733 = Subtract(x=w4919, y=w4918) -> (x-y=→"delay 78":u32)
            }
          }
          n1734 = call-dynamic "Read TelFocus.lvclass.vi"("error in (no error)"=w4897, "S4GUI in"=w4902) -> ("error out"=w4907:errorcluster, "TelFocus.lvclass"=w4908:refnum<class "TelFocus.lvclass">, "S4GUI out"=w4904:refnum<class "S4GUI.lvclass">)  [unwired: 7 in]
          n1735 = call-dynamic "Read SecMirror.lvclass.vi"("error in (no error)"=w4907, "TelFocus in"=w4908) -> ("error out"=w4876:errorcluster, "SecMirror.lvclass"=w4879:refnum<class "SecMirror.lvclass">, "TelFocus out"=w4906:refnum<class "TelFocus.lvclass">)  [unwired: 7 in]
          n1736 = call-dynamic "Read position.vi"("error in (no error)"=w4876, "SecMirror in"=w4879) -> ("error out"=w4875:errorcluster, "position"=w4872:i32, "SecMirror out"=w4878:refnum<class "SecMirror.lvclass">)  [unwired: 7 in]
          n1737 = call-dynamic "Read target.vi"("error in (no error)"=w4875, "SecMirror in"=w4878) -> ("error out"=w4874:errorcluster, "target"=w4873:i32, "SecMirror out"=w4877:refnum<class "SecMirror.lvclass">)  [unwired: 7 in]
          n1738 = Subtract(x=w4873, y=w4872) -> (x-y=w4871:i32)
          n1739 = Absolute Value(x=w4871) -> (abs(x)=w4870:i32)
          n1740 = call-dynamic "Read State Machine.vi"("error in (no error)"=w4874, "Device in"=w4877) -> ("error out"=w4887:errorcluster, "State Machine.lvclass"=w4890:refnum<class "State Machine.lvclass">, "Device out"=w4900:refnum<class "SecMirror.lvclass">)  [unwired: 7 in]
          n1741 = To Unsigned Long Integer(number=w4870) -> (unsigned 32bit integer=w4867:u32)
          n1742 = Add(x=w4867, y=u32 25000 ("period")) -> (x+y=w4868:u32)
          n1743 = call-dynamic "Verif Clock 2.vi"("error in (no error)"=w4887, "period (ms)"=w4868, "State Machine in"=w4890) -> ("error out"=w4886:errorcluster, "time elapsed"=→"time elapsed 2":u32, "State Machine out"=w4889:refnum<class "State Machine.lvclass">)  [unwired: 6 in]
          n1744 = call-dynamic "Read Timeout 2.vi"("error in (no error)"=w4886, "State Machine in"=w4889) -> ("error out"=w4885:errorcluster, "Timeout 2"=w4863:bool, "State Machine out"=w4888:refnum<class "State Machine.lvclass">)  [unwired: 7 in]
          n1745 = call-dynamic "Read State.vi"("error in (no error)"=w4885, "State Machine in"=w4888) -> ("error out"=w4895:errorcluster, "State"=w4866:i32, "State Machine out"=w4896:refnum<class "State Machine.lvclass">)  [unwired: 7 in]
          n1746 = Equal To 0?(x=w4866) -> (x = 0?=w4861:bool)
          n1747 = Equal?(x=w4866, y=90) -> (x = y?=w4864:bool)
          n1748 = call-dynamic "Write State Machine.vi"("error in (no error)"=w4895, "State Machine.lvclass"=w4896, "Device in"=w4900) -> ("error out"=w4899:errorcluster, "Device out"=w4901:refnum<class "SecMirror.lvclass">)  [unwired: 7 in]
          n1749 = call-dynamic "Write SecMirror.lvclass.vi"("error in (no error)"=w4899, "SecMirror.lvclass"=w4901, "TelFocus in"=w4906) -> ("error out"=w4903:errorcluster, "TelFocus out"=w4905:refnum<class "TelFocus.lvclass">)  [unwired: 7 in]
          n1750 = Or(x=w4864, y=w4863) -> (x .or. y?=w4862:bool)
          n1751 = call-dynamic "Write TelFocus.lvclass.vi"("error in (no error)"=w4903, "TelFocus.lvclass"=w4905, "S4GUI in"=w4904) -> ("error out"=w4892:errorcluster, "S4GUI out"=w4884:refnum<class "S4GUI.lvclass">)  [unwired: 7 in]
          n1752 = case shown="False" w4862 {
            tunnel: w4891 -> [w4911 _]
            tunnel: [w4911 u32 1 ("Obs_state")] -> w4881
            tunnel: w4884 -> [w4910 w4916]
            tunnel: [w4910 w4915] -> w4883
            tunnel: [w4909 FALSE] -> w4860
            tunnel: w4861 -> [w4909 _]
            frame False {
            }
            frame True {
              n1753 = Bundle By Name(cluster=w4916, "Error Msg"="ERROR: moving telescope focus timeout  (S4GUI:HandleObservationSync.vi - state 361)") -> (w4915:refnum<class "S4GUI.lvclass">)
            }
          }
          n1754 = Increment(x=w4881) -> (x+1=w4880:u32)
          n1755 = Select(t=w4880, s=w4860, f=w4881) -> (s? t:f=w4894:u32)
          n1756 = Bundle By Name(cluster=w4883, "Obs_state"=w4894) -> (w4893:refnum<class "S4GUI.lvclass">)
        }
        frame 362 {
          # "Envia dados para o header das imagens (Channel:Run.vi - estado 58)"
          n1757 = call-dynamic "Read AcquisitionA.vi"("error in (no error)"=w4962, "S4ACS_GUI in"=w4963) -> ("error out"=w4939:errorcluster, "Acquisition.lvclass"=w4942:refnum<class "Acquisition.lvclass">, "S4ACS_GUI out"=w4965:refnum<class "S4GUI.lvclass">)  [unwired: 7 in]
          n1758 = call-dynamic "Read enabled.vi"("error in (no error)"=w4939, "Server in"=w4942) -> ("error out"=w4938:errorcluster, "enabled"=w4940:bool, "Server out"=w4941:refnum<class "Acquisition.lvclass">)  [unwired: 7 in]
          n1759 = case shown="True" w4940 {
            tunnel: w4941 -> [w5021 w5036]
            tunnel: w4938 -> [w5020 w5035]
            tunnel: [w5021 w5033] -> w4966
            tunnel: [w5020 w5032] -> w4964
            frame False {
            }
            frame True {
              n1760 = call-dynamic "Read Channel.vi"("error in (no error)"=w5035, "Acquisition in"=w5036) -> ("error out"=w5028:errorcluster, "Channel.lvclass"=w5027:refnum<class "Channel.lvclass">, "Acquisition out"=w5034:refnum<class "Acquisition.lvclass">)  [unwired: 7 in]
              n1761 = call-dynamic "Read State Machine.vi"("error in (no error)"=w5028, "Device in"=w5027) -> ("error out"=w5029:errorcluster, "State Machine.lvclass"=w5031:refnum<class "State Machine.lvclass">, "Device out"=w5025:refnum<class "Channel.lvclass">)  [unwired: 7 in]
              n1762 = call "Next State.vi"("error in (no error)"=w5029, "New_State"=58, "State Machine in"=w5031) -> ("error out"=w5022:errorcluster, "State Machine out"=w5023:refnum<class "State Machine.lvclass">)  [unwired: 7 in]
              n1763 = call-dynamic "Write State Machine.vi"("error in (no error)"=w5022, "State Machine.lvclass"=w5023, "Device in"=w5025) -> ("error out"=w5024:errorcluster, "Device out"=w5026:refnum<class "Channel.lvclass">)  [unwired: 7 in]
              n1764 = call-dynamic "Write Channel.vi"("error in (no error)"=w5024, "Channel.lvclass"=w5026, "Acquisition in"=w5034) -> ("error out"=w5032:errorcluster, "Acquisition out"=w5033:refnum<class "Acquisition.lvclass">)  [unwired: 7 in]
            }
          }
          n1765 = call-dynamic "Write AcquisitionA.vi"("error in (no error)"=w4964, "Acquisition.lvclass"=w4966, "S4ACS_GUI in"=w4965) -> ("error out"=w4957:errorcluster, "S4ACS_GUI out"=w4958:refnum<class "S4GUI.lvclass">)  [unwired: 7 in]
          n1766 = call "Read AcquisitionB.vi"("error in (no error)"=w4957, "S4ACS_GUI in"=w4958) -> ("error out"=w4935:errorcluster, "Acquisition.lvclass"=w4937:refnum<class "Acquisition.lvclass">, "S4ACS_GUI out"=w4955:refnum<class "S4GUI.lvclass">)  [unwired: 7 in]
          n1767 = call-dynamic "Read enabled.vi"("error in (no error)"=w4935, "Server in"=w4937) -> ("error out"=w4934:errorcluster, "enabled"=w4933:bool, "Server out"=w4936:refnum<class "Acquisition.lvclass">)  [unwired: 7 in]
          n1768 = case shown="True" w4933 {
            tunnel: w4936 -> [w5004 w5019]
            tunnel: w4934 -> [w5003 w5018]
            tunnel: [w5004 w5016] -> w4956
            tunnel: [w5003 w5015] -> w4954
            frame False {
            }
            frame True {
              n1769 = call-dynamic "Read Channel.vi"("error in (no error)"=w5018, "Acquisition in"=w5019) -> ("error out"=w5011:errorcluster, "Channel.lvclass"=w5010:refnum<class "Channel.lvclass">, "Acquisition out"=w5017:refnum<class "Acquisition.lvclass">)  [unwired: 7 in]
              n1770 = call-dynamic "Read State Machine.vi"("error in (no error)"=w5011, "Device in"=w5010) -> ("error out"=w5012:errorcluster, "State Machine.lvclass"=w5014:refnum<class "State Machine.lvclass">, "Device out"=w5008:refnum<class "Channel.lvclass">)  [unwired: 7 in]
              n1771 = call "Next State.vi"("error in (no error)"=w5012, "New_State"=58, "State Machine in"=w5014) -> ("error out"=w5005:errorcluster, "State Machine out"=w5006:refnum<class "State Machine.lvclass">)  [unwired: 7 in]
              n1772 = call-dynamic "Write State Machine.vi"("error in (no error)"=w5005, "State Machine.lvclass"=w5006, "Device in"=w5008) -> ("error out"=w5007:errorcluster, "Device out"=w5009:refnum<class "Channel.lvclass">)  [unwired: 7 in]
              n1773 = call-dynamic "Write Channel.vi"("error in (no error)"=w5007, "Channel.lvclass"=w5009, "Acquisition in"=w5017) -> ("error out"=w5015:errorcluster, "Acquisition out"=w5016:refnum<class "Acquisition.lvclass">)  [unwired: 7 in]
            }
          }
          n1774 = call "Write AcquisitionB.vi"("error in (no error)"=w4954, "Acquisition.lvclass"=w4956, "S4ACS_GUI in"=w4955) -> ("error out"=w4950:errorcluster, "S4ACS_GUI out"=w4949:refnum<class "S4GUI.lvclass">)  [unwired: 7 in]
          n1775 = call-dynamic "Read AcquisitionC.vi"("error in (no error)"=w4950, "S4ACS_GUI in"=w4949) -> ("error out"=w4930:errorcluster, "Acquisition.lvclass"=w4932:refnum<class "Acquisition.lvclass">, "S4ACS_GUI out"=w4952:refnum<class "S4GUI.lvclass">)  [unwired: 7 in]
          n1776 = call-dynamic "Read enabled.vi"("error in (no error)"=w4930, "Server in"=w4932) -> ("error out"=w4929:errorcluster, "enabled"=w4928:bool, "Server out"=w4931:refnum<class "Acquisition.lvclass">)  [unwired: 7 in]
          n1777 = case shown="True" w4928 {
            tunnel: [w4986 w4994] -> w4953
            tunnel: [w4987 w4993] -> w4951
            tunnel: w4931 -> [w4987 w4991]
            tunnel: w4929 -> [w4986 w4990]
            frame False {
            }
            frame True {
              n1778 = call-dynamic "Read Channel.vi"("error in (no error)"=w4990, "Acquisition in"=w4991) -> ("error out"=w4998:errorcluster, "Channel.lvclass"=w4999:refnum<class "Channel.lvclass">, "Acquisition out"=w4992:refnum<class "Acquisition.lvclass">)  [unwired: 7 in]
              n1779 = call-dynamic "Read State Machine.vi"("error in (no error)"=w4998, "Device in"=w4999) -> ("error out"=w4997:errorcluster, "State Machine.lvclass"=w4995:refnum<class "State Machine.lvclass">, "Device out"=w5001:refnum<class "Channel.lvclass">)  [unwired: 7 in]
              n1780 = call "Next State.vi"("error in (no error)"=w4997, "New_State"=58, "State Machine in"=w4995) -> ("error out"=w4989:errorcluster, "State Machine out"=w4988:refnum<class "State Machine.lvclass">)  [unwired: 7 in]
              n1781 = call-dynamic "Write State Machine.vi"("error in (no error)"=w4989, "State Machine.lvclass"=w4988, "Device in"=w5001) -> ("error out"=w5002:errorcluster, "Device out"=w5000:refnum<class "Channel.lvclass">)  [unwired: 7 in]
              n1782 = call-dynamic "Write Channel.vi"("error in (no error)"=w5002, "Channel.lvclass"=w5000, "Acquisition in"=w4992) -> ("error out"=w4994:errorcluster, "Acquisition out"=w4993:refnum<class "Acquisition.lvclass">)  [unwired: 7 in]
            }
          }
          n1783 = call-dynamic "Write AcquisitionC.vi"("error in (no error)"=w4953, "Acquisition.lvclass"=w4951, "S4ACS_GUI in"=w4952) -> ("error out"=w4947:errorcluster, "S4ACS_GUI out"=w4946:refnum<class "S4GUI.lvclass">)  [unwired: 7 in]
          n1784 = call-dynamic "Read AcquisitionD.vi"("error in (no error)"=w4947, "S4ACS_GUI in"=w4946) -> ("error out"=w4925:errorcluster, "Acquisition.lvclass"=w4927:refnum<class "Acquisition.lvclass">, "S4ACS_GUI out"=w4945:refnum<class "S4GUI.lvclass">)  [unwired: 7 in]
          n1785 = call-dynamic "Read enabled.vi"("error in (no error)"=w4925, "Server in"=w4927) -> ("error out"=w4924:errorcluster, "enabled"=w4923:bool, "Server out"=w4926:refnum<class "Acquisition.lvclass">)  [unwired: 7 in]
          n1786 = case shown="True" w4923 {
            tunnel: w4924 -> [w4969 w4985]
            tunnel: [w4969 w4984] -> w4948
            tunnel: w4926 -> [w4970 w4975]
            tunnel: [w4970 w4973] -> w4944
            frame False {
            }
            frame True {
              n1787 = call-dynamic "Read Channel.vi"("error in (no error)"=w4985, "Acquisition in"=w4975) -> ("error out"=w4980:errorcluster, "Channel.lvclass"=w4979:refnum<class "Channel.lvclass">, "Acquisition out"=w4974:refnum<class "Acquisition.lvclass">)  [unwired: 7 in]
              n1788 = call-dynamic "Read State Machine.vi"("error in (no error)"=w4980, "Device in"=w4979) -> ("error out"=w4981:errorcluster, "State Machine.lvclass"=w4983:refnum<class "State Machine.lvclass">, "Device out"=w4977:refnum<class "Channel.lvclass">)  [unwired: 7 in]
              n1789 = call "Next State.vi"("error in (no error)"=w4981, "New_State"=58, "State Machine in"=w4983) -> ("error out"=w4971:errorcluster, "State Machine out"=w4972:refnum<class "State Machine.lvclass">)  [unwired: 7 in]
              n1790 = call-dynamic "Write State Machine.vi"("error in (no error)"=w4971, "State Machine.lvclass"=w4972, "Device in"=w4977) -> ("error out"=w4976:errorcluster, "Device out"=w4978:refnum<class "Channel.lvclass">)  [unwired: 7 in]
              n1791 = call-dynamic "Write Channel.vi"("error in (no error)"=w4976, "Channel.lvclass"=w4978, "Acquisition in"=w4974) -> ("error out"=w4984:errorcluster, "Acquisition out"=w4973:refnum<class "Acquisition.lvclass">)  [unwired: 7 in]
            }
          }
          n1792 = call-dynamic "Write AcquisitionD.vi"("error in (no error)"=w4948, "Acquisition.lvclass"=w4944, "S4ACS_GUI in"=w4945) -> ("error out"=w4922:errorcluster, "S4ACS_GUI out"=w4943:refnum<class "S4GUI.lvclass">)  [unwired: 7 in]
          n1793 = flat-sequence {
            tunnel: w4922 -> [w4967]
            tunnel: [w4967] -> w4921
            frame #0 {
              n1794 = Tick Count (ms)() -> (millisecond timer value=→"time9":u32)
            }
          }
          n1795 = Increment(x=w4961) -> (x+1=w4960:u32)
          n1796 = Bundle By Name(cluster=w4943, "Obs_state"=w4960) -> (w4959:refnum<class "S4GUI.lvclass">)
        }
        frame 363 {
          # "T: mode EXPOSE\nF: mode FIRE\nNa seq de foco, só \ndeve usar mode EXPOSE."
          # "Espera todos os canais chegarem ao estado de repouso.\n(estado 0  de Channel:Run.vi)."
          n1797 = call-dynamic "Read AcquisitionA.vi"("error in (no error)"=w5087, "S4ACS_GUI in"=w5088) -> ("error out"=w5066:errorcluster, "Acquisition.lvclass"=w5067:refnum<class "Acquisition.lvclass">, "S4ACS_GUI out"=w5090:refnum<class "S4GUI.lvclass">)  [unwired: 7 in]
          n1798 = call-dynamic "Read enabled.vi"("error in (no error)"=w5066, "Server in"=w5067) -> ("error out"=w5068:errorcluster, "enabled"=w5070:bool, "Server out"=w5069:refnum<class "Acquisition.lvclass">)  [unwired: 7 in]
          n1799 = case shown="True" w5070 {
            tunnel: [w5164 w5182] -> w5091
            tunnel: [w5163 w5181] -> w5089
            tunnel: w5069 -> [w5164 w5174]
            tunnel: w5068 -> [w5163 w5173]
            tunnel: [TRUE w5166] -> w5047
            tunnel: [FALSE w5167] -> w5043
            frame False {
            }
            frame True {
              n1800 = call-dynamic "Read Channel.vi"("error in (no error)"=w5173, "Acquisition in"=w5174) -> ("error out"=w5170:errorcluster, "Channel.lvclass"=w5171:refnum<class "Channel.lvclass">, "Acquisition out"=w5183:refnum<class "Acquisition.lvclass">)  [unwired: 7 in]
              n1801 = call-dynamic "Read wait_expose.vi"("error in (no error)"=w5170, "Channel in"=w5171) -> ("error out"=w5168:errorcluster, "wait_expose"=w5167:bool, "Channel out"=w5169:refnum<class "Channel.lvclass">)  [unwired: 7 in]
              n1802 = call-dynamic "Read State Machine.vi"("error in (no error)"=w5168, "Device in"=w5169) -> ("error out"=w5175:errorcluster, "State Machine.lvclass"=w5177:refnum<class "State Machine.lvclass">, "Device out"=w5179:refnum<class "Channel.lvclass">)  [unwired: 7 in]
              n1803 = call-dynamic "Read State.vi"("error in (no error)"=w5175, "State Machine in"=w5177) -> ("error out"=w5172:errorcluster, "State"=w5165:i32, "State Machine out"=w5176:refnum<class "State Machine.lvclass">)  [unwired: 7 in]
              n1804 = Equal To 0?(x=w5165) -> (x = 0?=w5166:bool)
              n1805 = call-dynamic "Write State Machine.vi"("error in (no error)"=w5172, "State Machine.lvclass"=w5176, "Device in"=w5179) -> ("error out"=w5178:errorcluster, "Device out"=w5180:refnum<class "Channel.lvclass">)  [unwired: 7 in]
              n1806 = call-dynamic "Write Channel.vi"("error in (no error)"=w5178, "Channel.lvclass"=w5180, "Acquisition in"=w5183) -> ("error out"=w5181:errorcluster, "Acquisition out"=w5182:refnum<class "Acquisition.lvclass">)  [unwired: 7 in]
            }
          }
          n1807 = call-dynamic "Write AcquisitionA.vi"("error in (no error)"=w5089, "Acquisition.lvclass"=w5091, "S4ACS_GUI in"=w5090) -> ("error out"=w5083:errorcluster, "S4ACS_GUI out"=w5084:refnum<class "S4GUI.lvclass">)  [unwired: 7 in]
          n1808 = call "Read AcquisitionB.vi"("error in (no error)"=w5083, "S4ACS_GUI in"=w5084) -> ("error out"=w5063:errorcluster, "Acquisition.lvclass"=w5065:refnum<class "Acquisition.lvclass">, "S4ACS_GUI out"=w5081:refnum<class "S4GUI.lvclass">)  [unwired: 7 in]
          n1809 = call-dynamic "Read enabled.vi"("error in (no error)"=w5063, "Server in"=w5065) -> ("error out"=w5062:errorcluster, "enabled"=w5061:bool, "Server out"=w5064:refnum<class "Acquisition.lvclass">)  [unwired: 7 in]
          n1810 = case shown="True" w5061 {
            tunnel: w5064 -> [w5141 w5160]
            tunnel: w5062 -> [w5140 w5159]
            tunnel: [w5141 w5157] -> w5082
            tunnel: [w5140 w5156] -> w5080
            tunnel: [TRUE w5148] -> w5046
            tunnel: [FALSE ("expose") w5142] -> w5042
            frame False {
            }
            frame True {
